vi "FPGA IO.vi"() -> ()   [LabVIEW 2014]
doc: "Accepts inputs from a host based VI for controlling analog and digital outputs on a R-series board containing an FPGA. This VI will produce 4 different signal types dependent on the user input and the channel of interest. When the <B>WaveType</B> is set to laser, the first three channels will produce either a sine or square wave at the frequency <B>f0</B> while the last two produce only square waves. When the wavetype is set to speaker or none, all channels produce the same signal (although for the speaker, signals with a gain of <B>Amp</B> applied)."
uses:
  Utilities/FPGA/Controls/FxdPt Props.ctl
  Reusable/PAS/Main/Controls/Laser Modulation.ctl
  <vilib>/Platform/TimedLoop/XDataNode/timing_clust.ctl
  <vilib>/Platform/TimedLoop/XDataNode/nitl_modes.ctl
  <vilib>/Platform/TimedLoop/XDataNode/wakeup.ctl
  <vilib>/rvi/Emulation/niFpgaGetClockAttributes.vi
  <vilib>/rvi/Emulation/niFpgaSctlEmulationGetInTimedLoop.vi
  <vilib>/rvi/Emulation/niFpgaEmulationReportErrorSimple.vi
  <vilib>/rvi/Emulation/niFpgaCriticalErrorInLSC.vi
  <vilib>/rvi/Emulation/niFpgaProcessEmulError.vi
  <vilib>/rvi/eio/common/nirviEmuTemplateMethod_errors.vi
  <vilib>/Platform/TimedLoop/XDataNode/XDataNode.xnode
  <vilib>/rvi/FXPMathLib/FxpMul/XNode/nifxpmath_Multiplier.xnode
  <vilib>/eio/EIONode/EIONode.xnode
  <vilib>/rvi/FXPMathLib/FxpAdd/XNode/nifxpmath_Add.xnode
  <vilib>/Platform/TimedLoop/XDataNode/XDNodeRunTimeDep.lvlib
  <vilib>/rvi/FXPMathLib/sim/FxpSim.dll
panel:
  in  "iSpk Enable":T1={"Ch1"=TRUE, "Ch2"=TRUE, "Ch3"=TRUE, "Ch4"=TRUE, "Ch5"=TRUE}
  in  "Speaker":cluster{"Voltage":fxp<+,14,1>, "Offset":i16}
  in  "Spk Enable":bool
  in  "LaserEn":T1
  in  "Cell 5":T2 {"Offset" format="%#.6f"; "Scale" format="%#.6f"}
  in  "Cell 4":T2 {"Offset" format="%#.6f"; "Scale" format="%#.6f"}
  in  "Cell 3":T2 {"Offset" format="%#.6f"; "Scale" format="%#.6f"}
  in  "Cell 2":T2 {"f0" format="%#.6g"; "Offset" format="%#.6f"; "Scale" format="%#.6f"}
  in  "Cell 1":T2 {"f0" format="%.0g"; "Offset" format="%#.6f"; "Scale" format="%#.6f"}
  out "Stopped":bool
  out "SquareOut":T4
  in  "stop":bool
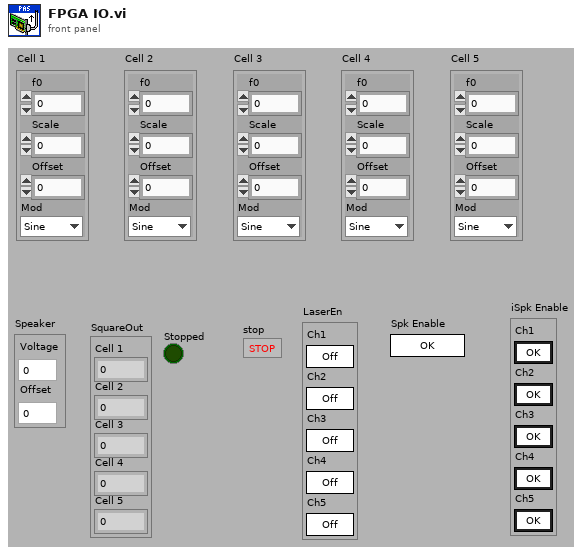
[diagram p1: front panel]
types:
  T1 = cluster{"Ch1":bool, "Ch2":bool, "Ch3":bool, "Ch4":bool, "Ch5":bool}
  T2 = typedef "FxdPt Props.ctl" = cluster{"f0":fxp<+,32,0>, "Scale":fxp<+,14,1>, "Offset":i16, "Mod":T3}
  T3 = typedef "Laser Modulation.ctl" = enum8{"Sine", "Square"}
  T4 = cluster{"Cell 1":i16, "Cell 2":i16, "Cell 3":i16, "Cell 4":i16, "Cell 5":i16}
  T5 = typedef "XDNodeRunTimeDep.lvlib/timing_clust.ctl" = cluster{"Expected End [f-1]":u64, "Actual End [f-1]":u64, "Finished Late? [f-1]":bool, "Expected End [i-1]":u64, "Actual End [i-1]":u64, "Finished Late? [i-1]":bool, "Expected Start [i]":u64, "Actual Start [i]":u64, "Expected Start [f]":u64, "Actual Start [f]":u64, "Source Name":string, "Structure Name":string, "Period":i64, "Deadline":i64, "Offset":i64, "Start":i64, "Priority":i32, "Timeout":i32, "Mode":T6, "Wakeup Reason":T7, "Error":errorcluster, "Source Type":string, "Secondary Source Type":string, "Global End Time":u64, "Global Start Time":u64, "Frame Duration":u64, "Iteration Duration":u64, "Assigned CPU":i32, "I/O Scan Engine Mode":u32}
  T6 = typedef "XDNodeRunTimeDep.lvlib/nitl_modes.ctl" = enum32{"No Change", "Process missed periods, maintain original phase", "Discard missed periods, maintain original phase", "Process missed periods, ignore original phase", "Discard missed periods, ignore original phase"}
  T7 = typedef "XDNodeRunTimeDep.lvlib/wakeup.ctl" = enum32{"Normal", "Aborted", "Asynchronous wakeup", "Timing source error", "Timed loop error", "Timeout"}
  T8 = cluster{"square wave out":i16, "square wave out":i16, "square wave out":i16, "square wave out":i16, "square wave out":i16}
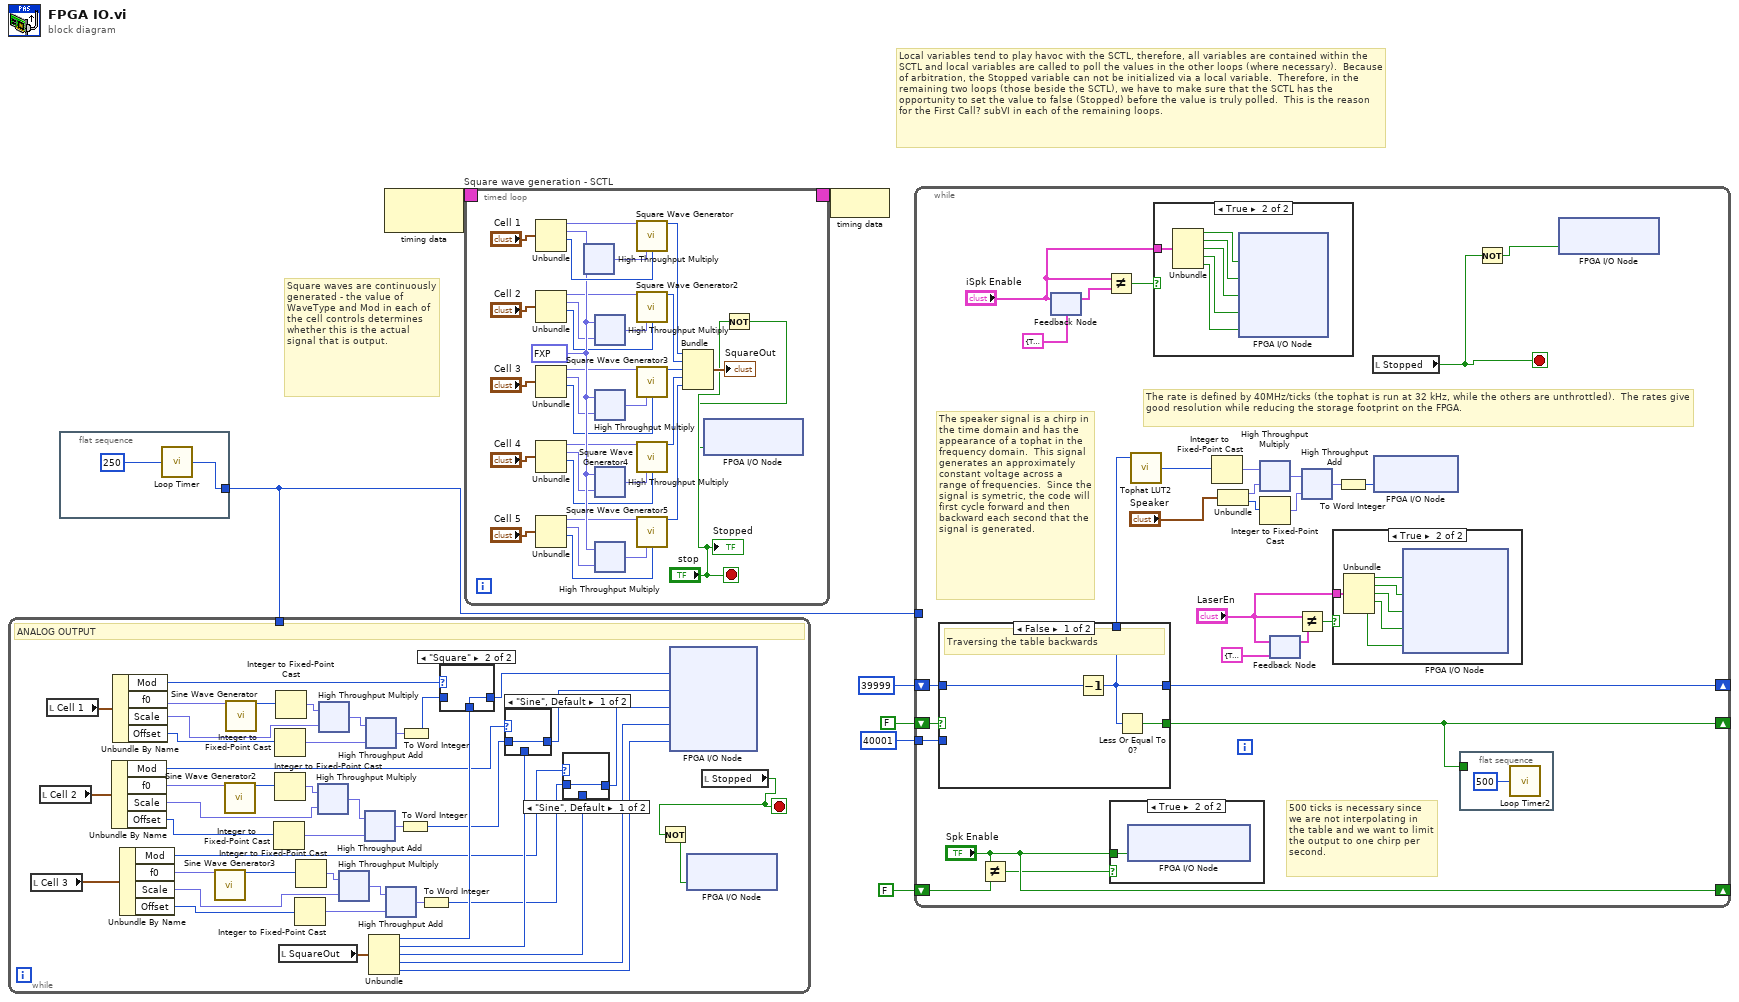
[diagram p0: block diagram]
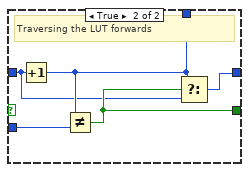
[diagram p5: hidden frame]
diagram:
  # "Square waves are continuously generated - the value of WaveType and Mod in each of the cell controls determines whether this is the actual signal that is output."
  # "Local variables tend to play havoc with the SCTL, therefore, all variables are contained within the SCTL and local variables are called to poll the values in the other loops (where necessary).  Because of arbitration, the Stopped variable can not be initialized via a local variable.  Therefore, in the remaining two loops (those beside the SCTL), we have to make sure that the SCTL has the opportunity to set the value to false (Stopped) before the value is truly polled.  This is the reason for the First Call? subVI in each of the remaining loops."
  n1 = while "Analog Output" {
    tunnel: w1 -> [_]
    stop <- w9 stop-if-true
    # "ANALOG OUTPUT"
    n2 = local read "Cell 3"() -> (w16:T2)
    n3 = local read "Cell 2"() -> (w17:T2)
    n4 = local read "Cell 1"() -> (w18:T2)
    n5 = Unbundle By Name(w17) -> ("Mod"=w11:T3, "f0"=w29:fxp<+,32,0>, "Scale"=w28:fxp<+,14,1>, "Offset"=w27:i16)
    n6 = Unbundle By Name(w18) -> ("Mod"=w12:T3, "f0"=w37:fxp<+,32,0>, "Scale"=w36:fxp<+,14,1>, "Offset"=w35:i16)
    n7 = Unbundle By Name(w16) -> ("Mod"=w10:T3, "f0"=w24:fxp<+,32,0>, "Scale"=w25:fxp<+,14,1>, "Offset"=w26:i16)
    n8 = call "Sine Wave Generator3"("frequency (periods/tick)"=w24) -> ("sine out"=w21:i16)  [unwired: 14 in]
    n9 = call "Sine Wave Generator2"("frequency (periods/tick)"=w29) -> ("sine out"=w32:i16)  [unwired: 14 in]
    n10 = call "Sine Wave Generator"("frequency (periods/tick)"=w37) -> ("sine out"=w40:i16)  [unwired: 14 in]
    n11 = Integer to Fixed-Point Cast(integer=w27) -> (fixed-point=w34:fxp<+/-,16,16>)  [unwired: 1 in]
    n12 = Integer to Fixed-Point Cast(integer=w35) -> (fixed-point=w38:fxp<+/-,16,16>)  [unwired: 1 in]
    n13 = Integer to Fixed-Point Cast(integer=w32) -> (fixed-point=w33:fxp<+/-,16,16>)  [unwired: 1 in]
    n14 = Integer to Fixed-Point Cast(integer=w40) -> (fixed-point=w39:fxp<+/-,16,16>)  [unwired: 1 in]
    n15 = local read "SquareOut"() -> (w46:T4)
    n16 = Integer to Fixed-Point Cast(integer=w26) -> (fixed-point=w19:fxp<+/-,16,16>)  [unwired: 1 in]
    n17 = Integer to Fixed-Point Cast(integer=w21) -> (fixed-point=w20:fxp<+/-,16,16>)  [unwired: 1 in]
    n18 = xnode ("High Throughput Multiply")("x"=w33, "y"=w28) -> ("x*y"=w30:fxp<+/-,30,17>)
    n19 = xnode ("High Throughput Multiply")("x"=w39, "y"=w36) -> ("x*y"=w42:fxp<+/-,30,17>)
    n20 = xnode ("High Throughput Multiply")("x"=w20, "y"=w25) -> ("x*y"=w23:fxp<+/-,30,17>)
    n21 = xnode ("High Throughput Add")("x"=w30, "y"=w34) -> ("x+y"=w31:fxp<+/-,16,16>)
    n22 = xnode ("High Throughput Add")("x"=w42, "y"=w38) -> ("x+y"=w41:fxp<+/-,16,16>)
    n23 = Unbundle(w46) -> ("Cell 1"=w45:i16, "Cell 2"=w44:i16, "Cell 3"=w43:i16, "Cell 4"=w48:i16, "Cell 5"=w47:i16)
    n24 = xnode ("High Throughput Add")("x"=w23, "y"=w19) -> ("x+y"=w22:fxp<+/-,16,16>)
    n25 = To Word Integer(number=w31) -> (16bit integer=w14:i16)
    n26 = To Word Integer(number=w41) -> (16bit integer=w15:i16)
    n27 = To Word Integer(number=w22) -> (16bit integer=w13:i16)
    n28 = case shown="\"Square\"" w12 {
      tunnel: w45 -> [_ w57]
      tunnel: [w56 w57] -> w51
      tunnel: w15 -> [w56 _]
      frame "Sine", Default {
      }
      frame "Square" {
      }
    }
    n29 = case shown="\"Sine\", Default" w11 {
      tunnel: w44 -> [_ w55]
      tunnel: [w54 w55] -> w50
      tunnel: w14 -> [w54 _]
      frame "Sine", Default {
      }
      frame "Square" {
      }
    }
    n30 = case shown="\"Sine\", Default" w10 {
      tunnel: w43 -> [_ w53]
      tunnel: [w52 w53] -> w49
      tunnel: w13 -> [w52 _]
      frame "Sine", Default {
      }
      frame "Square" {
      }
    }
    n31 = xnode "FPGA I/O Node"("Ch 1 AO"=w51, "Ch 2 AO"=w50, "Ch 3 AO"=w49, "Ch 4 AO"=w48, "Ch 5 AO"=w47) -> ()  [unwired: 5 in, 5 out]
    n32 = local read "Stopped"() -> (w9:bool)
    n33 = Not(x=w9) -> (.not. x?=w8:bool)
    n34 = xnode "FPGA I/O Node"("AO Loop"=w8) -> ()  [unwired: 1 in, 1 out]
  }
  n35 = flat-sequence {
    tunnel: [w58] -> w1
    frame #0 {
      n36 = call "Loop Timer"("Count(mSec)"=u32 250) -> ("Tick Count(mSec)"=w58:u32)
    }
  }
  n37 = node-c288() -> (w7:T5)  [unwired: 1 in]
  n38 = timed-loop "Square wave generation - SCTL" {
    timing: w7 -> [_]
    timing-out: [_] -> w6
    stop <- "stop" stop-if-true
    w82 = fxp<+,15,15> 32767.0 ("n")
    n39 = Unbundle("Cell 1") -> ("f0"=w85:fxp<+,32,0>, "Scale"=w84:fxp<+,14,1>, "Offset"=w83:i16)  [unwired: 1 out]
    n40 = Unbundle("Cell 2") -> ("f0"=w73:fxp<+,32,0>, "Scale"=w72:fxp<+,14,1>, "Offset"=w74:i16)  [unwired: 1 out]
    n41 = Unbundle("Cell 3") -> ("f0"=w70:fxp<+,32,0>, "Scale"=w71:fxp<+,14,1>, "Offset"=w75:i16)  [unwired: 1 out]
    n42 = Unbundle("Cell 4") -> ("f0"=w69:fxp<+,32,0>, "Scale"=w68:fxp<+,14,1>, "Offset"=w76:i16)  [unwired: 1 out]
    n43 = Unbundle("Cell 5") -> ("f0"=w63:fxp<+,32,0>, "Scale"=w62:fxp<+,14,1>, "Offset"=w77:i16)  [unwired: 1 out]
    n44 = xnode ("High Throughput Multiply")("x"=w84, "y"=w82) -> ("x*y"=w87:fxp<+,29,16>)
    n45 = xnode ("High Throughput Multiply")("x"=w82, "y"=w72) -> ("x*y"=w65:fxp<+,29,16>)
    n46 = xnode ("High Throughput Multiply")("x"=w82, "y"=w71) -> ("x*y"=w66:fxp<+,29,16>)
    n47 = xnode ("High Throughput Multiply")("x"=w82, "y"=w68) -> ("x*y"=w67:fxp<+,29,16>)
    n48 = xnode ("High Throughput Multiply")("x"=w82, "y"=w62) -> ("x*y"=w64:fxp<+,29,16>)
    n49 = call "Square Wave Generator"("frequency (periods/tick)"=w85, "amplitude"=w87, "offset"=w83) -> ("square wave out"=w93:i16)  [unwired: 12 in]
    n50 = call "Square Wave Generator2"("frequency (periods/tick)"=w73, "amplitude"=w65, "offset"=w74) -> ("square wave out"=w92:i16)  [unwired: 12 in]
    n51 = call "Square Wave Generator3"("frequency (periods/tick)"=w70, "amplitude"=w66, "offset"=w75) -> ("square wave out"=w91:i16)  [unwired: 12 in]
    n52 = call "Square Wave Generator4"("frequency (periods/tick)"=w69, "amplitude"=w67, "offset"=w76) -> ("square wave out"=w90:i16)  [unwired: 12 in]
    n53 = call "Square Wave Generator5"("frequency (periods/tick)"=w63, "amplitude"=w64, "offset"=w77) -> ("square wave out"=w89:i16)  [unwired: 12 in]
    n54 = Bundle("square wave out"=w93, "square wave out"=w92, "square wave out"=w91, "square wave out"=w90, "square wave out"=w89) -> (→"SquareOut":T8)  [unwired: 1 in]
    n55 = Not(x="stop") -> (.not. x?=w60:bool)
    n56 = xnode "FPGA I/O Node"("SQW Loop"=w60) -> ()  [unwired: 1 in, 1 out]
    "Stopped" <- "stop"
  }
  n57 = node-c288(w6) -> ()
  n58 = while {
    shift-right: [w102] -> _
    shift-left: FALSE -> [w123]
    shift-right: [w103] -> _
    shift-left: u16 39999 -> [w104]
    shift-right: ["Spk Enable"] -> _
    shift-left: FALSE ("Spk Enable") -> [w116]
    tunnel: u16 40001 ("y") -> [w105]
    tunnel: w1 -> [_]
    stop <- w97 stop-if-true
    # "The rate is defined by 40MHz/ticks (the tophat is run at 32 kHz, while the others are unthrottled).  The rates give good resolution while reducing the storage footprint on the FPGA."
    # "500 ticks is necessary since we are not interpolating in the table and we want to limit the output to one chirp per second."
    # "The speaker signal is a chirp in the time domain and has the appearance of a tophat in the frequency domain.  This signal generates an approximately constant voltage across a range of frequencies.  Since the signal is symetric, the code will first cycle forward and then backward each second that the signal is generated."
    n59 = case "Check where we are in the chirp" shown="False" w123 {
      tunnel: w104 -> [w140 w141]
      tunnel: [w139 w144] -> w102
      tunnel: [w138 w145] -> w114
      tunnel: w105 -> [_ w143]
      tunnel: [w138 w142] -> w103
      frame False {
        # "Traversing the table backwards"
        n60 = Decrement(x=w140) -> (x-1=w138:u16)
        n61 = Less Or Equal To 0?(x=w138) -> (x <= 0?=w139:bool)
      }
      frame True {
        # "Traversing the LUT forwards"
        n62 = Increment(x=w141) -> (x+1=w145:u16)
        n63 = Not Equal?(x=w145, y=w143) -> (x != y?=w144:bool)
        n64 = Select(t=w145, s=w144, f=w141) -> (s? t:f=w142:u16)
      }
    }
    n65 = Not Equal?(x="Spk Enable", y=w116) -> (x != y?=w115:bool)
    n66 = feedback #1(T1 {"Ch1"=TRUE, "Ch2"=TRUE, "Ch3"=TRUE, "Ch4"=TRUE, "Ch5"=TRUE} ("iSpk Enable")) -> (w101:T1)
    n67 = feedback-in #1("iSpk Enable") -> ()
    n68 = Not Equal?(x="iSpk Enable", y=w101) -> (x != y?=w99:bool)
    n69 = case shown="True" w115 {
      tunnel: "Spk Enable" -> [_ w137]
      frame False {
      }
      frame True {
        n70 = xnode "FPGA I/O Node"("Speaker Enable"=w137) -> ()  [unwired: 1 in, 1 out]
      }
    }
    n71 = call "Tophat LUT2"("address"=w114) -> ("data out"=w120:i16)  [unwired: 8 in]
    n72 = case shown="True" w99 {
      tunnel: "iSpk Enable" -> [_ w129]
      frame False {
      }
      frame True {
        n73 = Unbundle(w129) -> ("Ch1"=w128:bool, "Ch2"=w127:bool, "Ch3"=w126:bool, "Ch4"=w125:bool, "Ch5"=w124:bool)
        n74 = xnode "FPGA I/O Node"("Spk Sel 2"=w128, "Spk Sel 1"=w127, "Spk Sel 3"=w126, "Spk Sel 4"=w125, "Spk Sel 5"=w124) -> ()  [unwired: 5 in, 5 out]
      }
    }
    n75 = Integer to Fixed-Point Cast(integer=w120) -> (fixed-point=w119:fxp<+/-,16,16>)  [unwired: 1 in]
    n76 = Unbundle("Speaker") -> ("Voltage"=w108:fxp<+,14,1>, "Offset"=w107:i16)
    n77 = xnode ("High Throughput Multiply")("x"=w119, "y"=w108) -> ("x*y"=w122:fxp<+/-,30,17>)
    n78 = Integer to Fixed-Point Cast(integer=w107) -> (fixed-point=w121:fxp<+/-,16,16>)  [unwired: 1 in]
    n79 = feedback #2(T1 {"Ch1"=TRUE, "Ch2"=TRUE, "Ch3"=TRUE, "Ch4"=TRUE, "Ch5"=TRUE} ("LaserEn")) -> (w109:T1)
    n80 = feedback-in #2("LaserEn") -> ()
    n81 = Not Equal?(x="LaserEn", y=w109) -> (x != y?=w111:bool)
    n82 = xnode ("High Throughput Add")("x"=w122, "y"=w121) -> ("x+y"=w113:fxp<+/-,31,18>)
    n83 = case shown="True" w111 {
      tunnel: "LaserEn" -> [_ w136]
      frame False {
      }
      frame True {
        n84 = Unbundle(w136) -> ("Ch1"=w135:bool, "Ch2"=w134:bool, "Ch3"=w133:bool, "Ch4"=w132:bool, "Ch5"=w131:bool)
        n85 = xnode "FPGA I/O Node"("Ch 1 Enable"=w135, "Ch 2 Enable"=w134, "Ch 3 Enable"=w133, "Ch 4 Enable"=w132, "Ch 5 Enable"=w131) -> ()  [unwired: 5 in, 5 out]
      }
    }
    n86 = To Word Integer(number=w113) -> (16bit integer=w118:i16)
    n87 = local read "Stopped"() -> (w97:bool)
    n88 = xnode "FPGA I/O Node"("Speaker"=w118) -> ()  [unwired: 1 in, 1 out]
    n89 = flat-sequence {
      tunnel: w102 -> [_]
      frame #0 {
        n90 = call "Loop Timer2"("Count(Ticks)"=u32 500) -> ()  [unwired: 1 out]
      }
    }
    n91 = Not(x=w97) -> (.not. x?=w96:bool)
    n92 = xnode "FPGA I/O Node"("Main Loop"=w96) -> ()  [unwired: 1 in, 1 out]
  }
